vi "Save multiple images to new tiff stack.vi"(7 "Compression Type (None)":i32(ring) items=["None", "JPEG", "Run Length Encoded", "Zip"], 8 "error in":errorcluster, 10 "Array of Images (U8, U16, I16)":T1[](array[typedef]), 11 "Path":path) -> (0 "error out":errorcluster)   [LabVIEW 2015]
doc: "This .vi saves an array of images into a new single .tiff stack file."
uses:
  Tiff reader.lvlib
  <vilib>/vision/Image Controls.llb/IMAQ Image.ctl
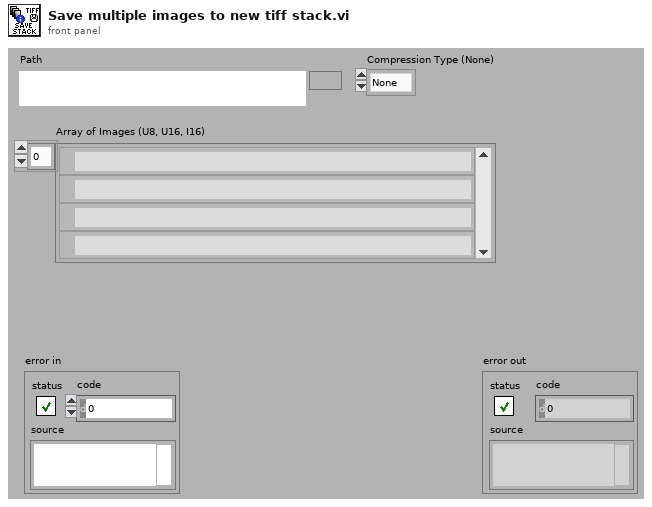
[diagram p1: front panel]
types:
  T1 = typedef "IMAQ Image.ctl" = refnum<image>
  T2 = cluster{"Rows Per Strip":i32, "Photometric":i32, "Compression Type":i32}
  T3 = typedef "Image Type" = u32
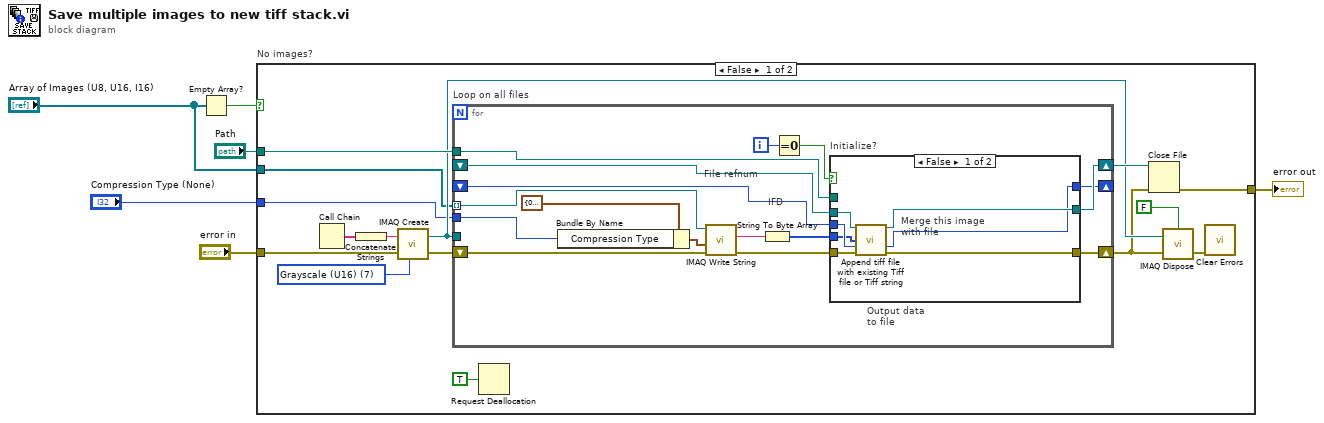
[diagram p0: block diagram]
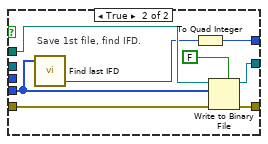
[diagram p2: hidden frame]
diagram:
  n1 = Empty Array?(array="Array of Images (U8, U16, I16)") -> (empty?=w2:bool)
  n2 = case "No images?" shown="False" w2 {
    tunnel: "Array of Images (U8, U16, I16)" -> [w15 _]
    tunnel: [w7 w53] -> w5
    tunnel: "error in" -> [w8 w53]
    tunnel: "Path" -> [w19 _]
    tunnel: "Compression Type (None)" -> [w11 _]
    frame False {
      w18 = T3 7 items=["Grayscale (U8)", "Grayscale (I16)", "Grayscale (SGL)", "Complex (CSG)", "RGB (U32)", "HSL (U32)", "RGB (U64)", "Grayscale (U16)"] ("Image Type")
      n3 = Call Chain() -> (call chain=w13:string[])
      n4 = Concatenate Strings(w13) -> (w12:string)
      n5 = call "IMAQ Create"("Image Name"=w12, "Image Type"=w18, "error in (no error)"=w8) -> ("New Image"=w16:T1, "error out"=w17:errorcluster)  [unwired: 1 in, 1 out]
      n6 = for "Loop on all files" {
        tunnel: w15 -> [w29] mode=indexing
        tunnel: w19 -> [w36]
        shift-right: [w35] -> w14
        shift-left: w17 -> [w30]
        shift-right: [w34] -> w20
        shift-left: _ -> [w33]
        shift-right: [w31] -> _
        shift-left: _ -> [w32]
        tunnel: w16 -> [_]
        tunnel: w11 -> [w26]
        i -> [w25]
        # "File refnum"
        # "IFD"
        # "Output data\nto file"
        n7 = Bundle By Name(cluster=T2 {"Rows Per Strip"=0, "Photometric"=1, "Compression Type"=0} ("TIFF Options"), "Compression Type"=w26) -> (w23:T2)
        n8 = call-poly "IMAQ Write String"("error in (no error)"=w30, "TIFF Options"=w23, "Image"=w29) -> ("error out"=w28:errorcluster, "FileString"=w22:string)  [unwired: 2 in, 5 out]
        n9 = String To Byte Array(string=w22) -> (unsigned byte array=w27:u8[])
        n10 = Equal To 0?(x=w25) -> (x = 0?=w37:bool)
        n11 = case "Initialize?" shown="False" w37 {
          tunnel: w28 -> [w43 w48]
          tunnel: w36 -> [_ w49]
          tunnel: [w44 w52] -> w35
          tunnel: [w41 w51] -> w34
          tunnel: w33 -> [w42 _]
          tunnel: w32 -> [w40 _]
          tunnel: [w39 w46] -> w31
          tunnel: w27 -> [w38 w45]
          frame False {
            # "Merge this image\nwith file"
            n12 = call "Append tiff file with existing Tiff file or Tiff string.vi"("Existing Tiff File (A) refnum"=w42, "Tiff file (B)\n (unsigned byte array)"=w38, "Location in existing file of\nit's last page's \n\"next IFD pointer\""=w40, "error in"=w43) -> ("File refnum out"=w41:refnum<file>, "Location in new file of\nit's last page's \n\"next IFD pointer\""=w39:i64, "error out"=w44:errorcluster)  [unwired: 3 in, 6 out]
          }
          frame True {
            # "Save 1st file, find IFD."
            n13 = call "Find last IFD.vi"("TIFF Data in"=w45) -> ("Location in byte stream of last IFD pointer.  This\nis the word to change if you are adding another page\nto the file."=w47:i32)  [unwired: 4 out]
            n14 = To Quad Integer(1:w47) -> (0:w46:i64)
            n15 = Write to Binary File(file (use dialog)=w49, data=w45, error in=w48, 5:FALSE ("prepend array or string size? (T)")) -> (refnum out=w51:refnum<file>, error out=w52:errorcluster)  [unwired: 1 in, 2 out]
          }
        }
      }
      n16 = Request Deallocation(TRUE ("flag")) -> ()
      n17 = Close File(refnum=w20, error in=w14) -> (error out=w7:errorcluster)  [unwired: 1 out]
      n18 = call "IMAQ Dispose"("All Images? (No)"=FALSE, "Image"=w16, "error in (no error)"=w14) -> ("error out"=w21:errorcluster)  [unwired: 3 out]
      n19 = call <vilib>:"Clear Errors.vi"("error in (no error)"=w21) -> ()  [unwired: 1 in, 6 out]
    }
    frame True {
    }
  }
  "error out" <- w5
